vi "ThousandSons.vi"() -> ()   [LabVIEW 2016]
panel:
  out "concatenated string":string
  in  "Numeric":i32
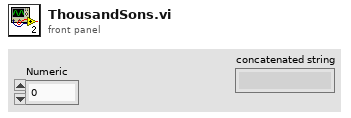
[diagram p1: front panel]
types:
  T1 = cluster{"Start":cluster{"X":dbl, "Y":dbl, "Z":dbl}, "End":cluster{"X":dbl, "Y":dbl, "Z":dbl}, "dir":string}
  T2 = cluster{"Start":cluster{"X":dbl, "Y":dbl, "Z":dbl}, "End":cluster{"X":dbl, "Y":dbl, "Z":dbl}, "dir":string}[]
  T3 = enum16{"open", "replace", "create", "open or create", "replace or create", "replace or create with confirmation"}
  T4 = typedef "IMAQ Image.ctl" = refnum<image>
  T5 = typedef "ControllerDiagPacket.ctl" = cluster{"Number of Diag Packets":i32, "Axes":T6[], "error":errorcluster}
  T6 = typedef "AxisDiagPacket.ctl" = cluster{"Axis Name":string, "Analog Input 0":dbl, "Analog Input 1":dbl, "Axis Fault (num)":i32, "Axis Fault (str)":string, "Axis Fault (bits)":cluster{"AmplifierFault":bool, "AmplifierTemperatureFault":bool, "CcwEndOfTravelLimitFault":bool, "CcwSoftwareLimitFault":bool, "CommunicationLostFault":bool, "CwEndOfTravelLimitFault":bool, "CwSoftwareLimitFault":bool, "EmergencyStopFault":bool, "EncoderFault":bool, "ExternalFault":bool, "FeedbackScalingFault":bool, "GantryMisalignFault ":bool, "HallSensorFault":bool, "InPositionTimeoutFault":bool, "InternalFault":bool, "MarkerSearchFault":bool, "MaxVelocityCommandFault":bool, "MissedInterruptFault":bool, "MotorTemperatureFault":bool, "None":bool, "OverCurrentFault":bool, "PositionErrorFault":bool, "PositionFeedbackFault":bool, "PowerSupplyFault":bool, "ProbeInputFault":bool, "SafeZoneFault":bool, "VelocityErrorFault":bool, "VelocityFeedbackFault":bool, "VoltageClampFault":bool}, "Axis Status (num)":i32, "Axis Status (str)":string, "Axis Status (bits)":cluster{"BacklashActive":bool, "CalibrationEnabled1D":bool, "CalibrationEnabled2D":bool, "CommandValid":bool, "DriveAbortPending":bool, "DrivePending":bool, "Enabling":bool, "GainMappingEnabled":bool, "GantryAligned":bool, "GantryRealigning":bool, "Homed":bool, "Homing":bool, "IFOVEnabled":bool, "JogGenerating":bool, "Jogging":bool, "JoystickControl":bool, "MasterSlaveControl":bool, "MotionBlocked":bool, "MotionClamped":bool, "MoveDone":bool, "None":bool, "NotVirtual":bool, "Profiling":bool, "Stability0":bool, "Stability1":bool, "TrajectoryFiltering":bool, "WaitDone":bool}, "Current Command":sgl, "Current Error":sgl, "Current Feedback":sgl, "Digital Inputs":i32, "Digital Outputs":i32, "Drive Status":i32, "Drive Status (str)":string, "Drive Status (bits)":cluster{"AccelerationPhase":bool, "AutofocusActive":bool, "BrakeOutput":bool, "CcwEndOfTravelLimitInput":bool, "CosineEncoderError":bool, "CurrentClamp":bool, "CwEndOfTravelLimitInput":bool, "DecelerationPhase":bool, "DualLoopActive":bool, "EmergencyStopInput":bool, "Enabled":bool, "EncoderClipping":bool, "GalvoCalibrationEnabled":bool, "GalvoPowerCorrection":bool, "HallAInput":bool, "HallBInput":bool, "HallCInput":bool, "HighResolutionMode":bool, "HomeLimitInput":bool, "InPosition":bool, "InPosition2":bool, "MarkerInput":bool, "MarkerLatch":bool, "MoveActive":bool, "NoMotorSupply":bool, "None":bool, "PowerLimiting":bool, "ProgrammingFlash":bool, "ProgrammingMXH":bool, "PSOHaltLatch":bool, "ServoControl":bool, "SineEncoderError":bool}, "Position Feedback Auxiliary":dbl, "Position Command":dbl, "Position Error":dbl, "Position Feedback":dbl, "Program Position Command":dbl, "Program Position Error":dbl, "Program Position Feedback":dbl, "Velocity Command":dbl, "Velocity Error":dbl, "Velocity Feedback":dbl}
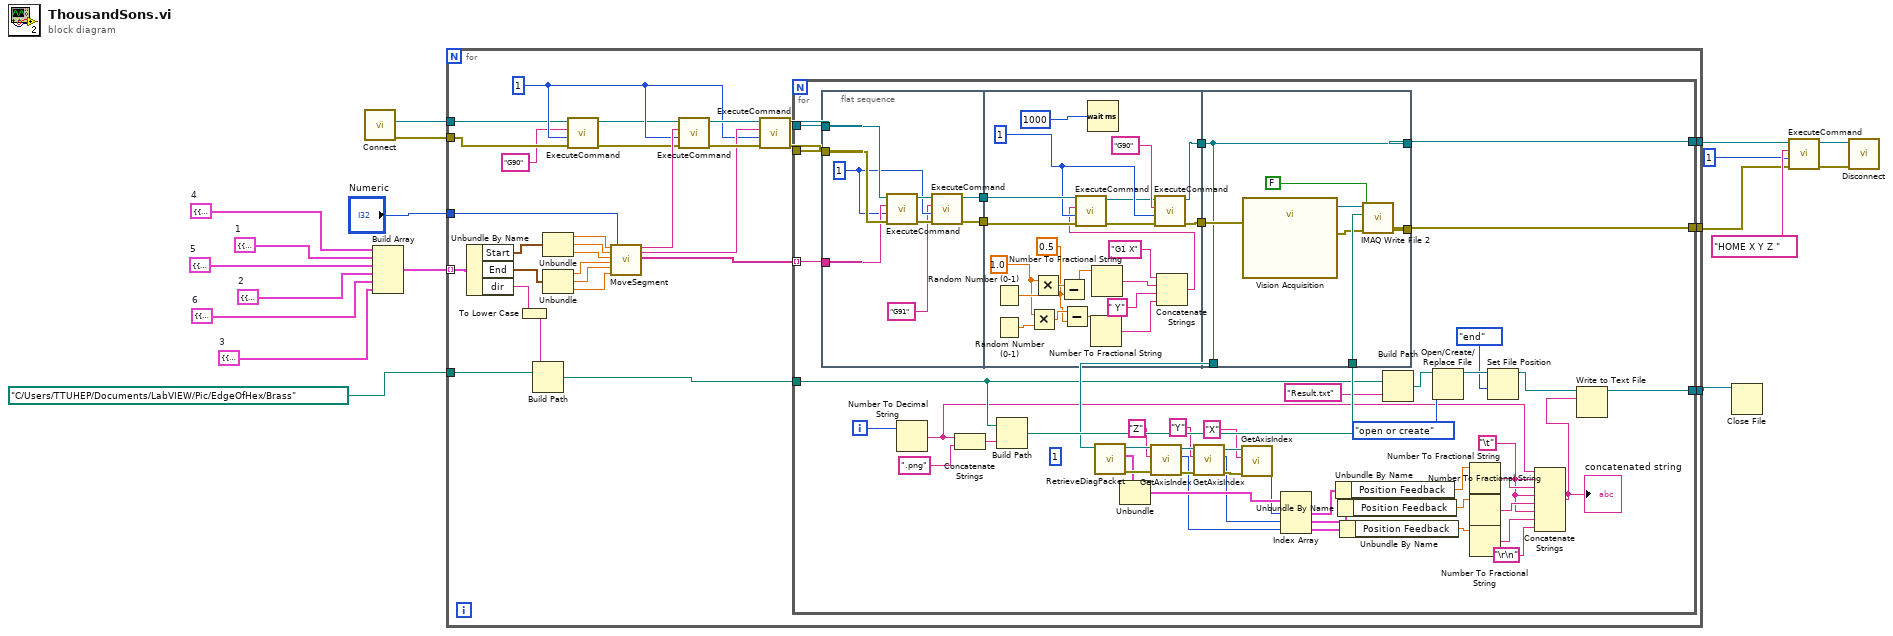
[diagram p0: block diagram]
diagram:
  w2 = T1 {"Start"={"X"=780.25388, "Y"=1006.48079, "Z"=72.88297}, "End"={"X"=744.18075, "Y"=1067.5354, "Z"=73.0907}, "dir"="sixth"}  # 6
  w4 = T1 {"Start"={"X"=655.48194, "Y"=913.5752, "Z"=72.84929}, "End"={"X"=728.37725, "Y"=914.09127, "Z"=72.91912}, "dir"="fifth"}  # 5
  w6 = T1 {"Start"={"X"=638.02499, "Y"=1067.21926, "Z"=72.79612}, "End"={"X"=602.49624, "Y"=1004.51285, "Z"=72.91934}, "dir"="forth"}  # 4
  w18 = T1 {"Start"={"X"=728.97095, "Y"=1077.84094, "Z"=72.8824}, "End"={"X"=652.4722, "Y"=1077.18423, "Z"=72.86214}, "dir"="third"}  # 3
  w3 = T1 {"Start"={"X"=743.14731, "Y"=921.06701, "Z"=72.79405}, "End"={"X"=782.17961, "Y"=989.61189, "Z"=72.90896}, "dir"="second"}  # 2
  w5 = T1 {"Start"={"X"=600.16895, "Y"=989.48771, "Z"=72.8227}, "End"={"X"=640.75654, "Y"=920.71587, "Z"=72.83136}, "dir"="first"}  # 1
  n1 = call "Connect.vi"() -> ("error out"=w15:errorcluster, "controller"=w14:refnum<k24>)  [unwired: 10 in]
  n2 = Build Array(w6, w5, w4, w3, w2, w18) -> (w17:T2)
  n3 = for {
    tunnel: w17 -> [w34] mode=indexing
    tunnel: "Numeric" -> [w42]
    tunnel: w15 -> [w24]
    tunnel: w14 -> [w26]
    tunnel: path "C:/Users/TTUHEP/Documents/LabVIEW/Pic/EdgeOfHex/Brass" -> [w31]
    tunnel: [w29] -> w12
    tunnel: [w28] -> w9
    tunnel: [w19] -> w1
    w27 = 1
    n4 = Unbundle By Name(w34) -> ("Start"=w33:cluster{"X":dbl, "Y":dbl, "Z":dbl}, "End"=w32:cluster{"X":dbl, "Y":dbl, "Z":dbl}, "dir"=w21:string)
    n5 = To Lower Case(string=w21) -> (all lower case string=w20:string)
    n6 = Build Path(base path=w31, name or relative path=w20) -> (appended path=w30:path)
    n7 = Unbundle(w33) -> ("X"=w48:dbl, "Y"=w47:dbl, "Z"=w46:dbl)
    n8 = Unbundle(w32) -> ("X"=w45:dbl, "Y"=w44:dbl, "Z"=w43:dbl)
    n9 = call "ExecuteCommand.vi"("error in (no error)"=w24, "taskId"=w27, "Command Code"="G90", "controller in"=w26) -> ("error out"=w23:errorcluster, "controller out"=w25:refnum<k24>)  [unwired: 5 in, 1 out]
    n10 = call "MoveSegment.vi"("Start X"=w48, "Start Y"=w47, "Start Z"=w46, "End X"=w45, "End Y"=w44, "End Z"=w43, "Number"=w42) -> ("Comm1"=w39:string, "Comm2"=w38:string, "Comm"=w35:string[])  [unwired: 10 in]
    n11 = call "ExecuteCommand.vi"("error in (no error)"=w23, "taskId"=w27, "Command Code"=w39, "controller in"=w25) -> ("error out"=w41:errorcluster, "controller out"=w40:refnum<k24>)  [unwired: 5 in, 1 out]
    n12 = call "ExecuteCommand.vi"("error in (no error)"=w41, "taskId"=w27, "Command Code"=w38, "controller in"=w40) -> ("error out"=w37:errorcluster, "controller out"=w36:refnum<k24>)  [unwired: 5 in, 1 out]
    n13 = for {
      tunnel: w37 -> [w93]
      tunnel: w36 -> [w92]
      tunnel: w35 -> [w94] mode=indexing
      tunnel: w30 -> [w58]
      tunnel: [w87] -> w29
      tunnel: [w86] -> w28
      tunnel: [w52] -> w19
      i -> [w97]
      w49 = "\t"
      (unwired) 1
      n14 = flat-sequence {
        tunnel: w94 -> [w104]
        tunnel: w93 -> [w105]
        tunnel: w92 -> [w106]
        tunnel: [w101] -> w91
        tunnel: [w100] -> w90
        tunnel: w91 -> [w128]
        tunnel: w90 -> [w127]
        tunnel: [w118] -> w88
        tunnel: [w122] -> w85
        tunnel: w89 -> [w134]
        tunnel: w88 -> [w129]
        tunnel: [w129] -> w87
        tunnel: [w131] -> w86
        tunnel: w85 -> [w130]
        tunnel: [w129] -> w84
        frame #0 {
          w99 = 1
          n15 = call "ExecuteCommand.vi"("error in (no error)"=w105, "taskId"=w99, "Command Code"=w104, "controller in"=w106) -> ("error out"=w103:errorcluster, "controller out"=w102:refnum<k24>)  [unwired: 5 in, 1 out]
          n16 = call "ExecuteCommand.vi"("error in (no error)"=w103, "taskId"=w99, "Command Code"="G91", "controller in"=w102) -> ("error out"=w100:errorcluster, "controller out"=w101:refnum<k24>)  [unwired: 5 in, 1 out]
        }
        frame #1 {
          w107 = 0.5
          w124 = 1.0
          w121 = 1
          n17 = Random Number (0-1)() -> (number: 0 to 1=w126:dbl)
          n18 = Random Number (0-1)() -> (number: 0 to 1=w125:dbl)
          n19 = Multiply(x=w124, y=w125) -> (x*y=w108:dbl)
          n20 = Multiply(x=w124, y=w126) -> (x*y=w111:dbl)
          n21 = Subtract(x=w111, y=w107) -> (x-y=w109:dbl)
          n22 = Subtract(x=w108, y=w107) -> (x-y=w110:dbl)
          n23 = Wait (ms)(milliseconds to wait=1000) -> ()  [unwired: 1 out]
          n24 = Number To Fractional String(number=w110) -> (F-format string=w114:string)  [unwired: 3 in]
          n25 = Number To Fractional String(number=w109) -> (F-format string=w116:string)  [unwired: 3 in]
          n26 = Concatenate Strings("G1 X", w116, " Y", w114) -> (w113:string)
          n27 = call "ExecuteCommand.vi"("error in (no error)"=w127, "taskId"=w121, "Command Code"=w113, "controller in"=w128) -> ("error out"=w123:errorcluster, "controller out"=w119:refnum<k24>)  [unwired: 5 in, 1 out]
          n28 = call "ExecuteCommand.vi"("error in (no error)"=w123, "taskId"=w121, "Command Code"="G90", "controller in"=w119) -> ("error out"=w122:errorcluster, "controller out"=w118:refnum<k24>)  [unwired: 5 in, 1 out]
        }
        frame #2 {
          n29 = call "Vision Acquisition"("error in"=w130) -> ("Image Out"=w135:T4, "error out"=w133:errorcluster)  [unwired: 25 in]
          n30 = call-poly "IMAQ Write File 2"("error in (no error)"=w133, "Compress? (N)"=FALSE, "File Path"=w134, "Image"=w135) -> ("error out"=w131:errorcluster)  [unwired: 6 in, 1 out]
        }
      }
      n31 = Number To Decimal String(number=w97) -> (decimal integer string=w50:string)  [unwired: 1 in]
      n32 = Concatenate Strings(w50, ".png") -> (w95:string)
      n33 = Build Path(base path=w58, name or relative path=w95) -> (appended path=w89:path)
      n34 = call "RetrieveDiagPacket.vi"("Controller In"=w84) -> ("error out"=w83:errorcluster, "ControllerDiagPacket"=w77:T5, "Controller Out"=w82:refnum<k24>)  [unwired: 8 in]
      n35 = Unbundle(w77) -> ("Axes"=w76:T6[])  [unwired: 2 out]
      n36 = call "GetAxisIndex.vi"("error in (no error)"=w83, "axis name"="Z", "controller in"=w82) -> ("error out"=w81:errorcluster, "axis index"=w75:i32, "controller out"=w80:refnum<k24>)  [unwired: 6 in]
      n37 = call "GetAxisIndex.vi"("error in (no error)"=w81, "axis name"="Y", "controller in"=w80) -> ("error out"=w79:errorcluster, "axis index"=w74:i32, "controller out"=w78:refnum<k24>)  [unwired: 6 in]
      n38 = call "GetAxisIndex.vi"("error in (no error)"=w79, "axis name"="X", "controller in"=w78) -> ("axis index"=w73:i32)  [unwired: 6 in, 2 out]
      n39 = Index Array(array=w76, index #1=w73, index #2=w74, index #3=w75) -> (element #1=w69:T6, element #2=w68:T6, element #3=w67:T6)
      n40 = Unbundle By Name(w69) -> ("Position Feedback"=w66:dbl)
      n41 = Unbundle By Name(w68) -> ("Position Feedback"=w65:dbl)
      n42 = Unbundle By Name(w67) -> ("Position Feedback"=w64:dbl)
      n43 = Build Path(base path=w58, name or relative path="Result.txt") -> (appended path=w57:path)
      n44 = Open/Create/Replace File(file path (use dialog)=w57, operation (0:open)=T3."open or create") -> (refnum out=w56:refnum<file>)  [unwired: 4 in, 2 out]
      n45 = Number To Fractional String(number=w66) -> (F-format string=w63:string)  [unwired: 3 in]
      n46 = Number To Fractional String(number=w65) -> (F-format string=w62:string)  [unwired: 3 in]
      n47 = Number To Fractional String(number=w64) -> (F-format string=w61:string)  [unwired: 3 in]
      n48 = Set File Position(refnum=w56, from (0:start)=enum16{"start", "end", "current"}."end") -> (refnum out=w55:refnum<file>)  [unwired: 2 in, 1 out]
      n49 = Concatenate Strings(w50, w49, w63, w49, w62, w49, w61, "\r\n") -> (w59:string)
      "concatenated string" <- w59
      n50 = Write to Text File(file (use dialog)=w55, text=w59) -> (refnum out=w52:refnum<file>)  [unwired: 2 in, 2 out]
    }
  }
  n51 = Close File(refnum=w1) -> ()  [unwired: 1 in, 2 out]
  n52 = call "ExecuteCommand.vi"("error in (no error)"=w9, "taskId"=1, "Command Code"="HOME X Y Z ", "controller in"=w12) -> ("error out"=w7:errorcluster, "controller out"=w8:refnum<k24>)  [unwired: 5 in, 1 out]
  n53 = call "Disconnect.vi"("error in (no error)"=w7, "controller"=w8) -> ()  [unwired: 9 in, 1 out]
